vi "Load Core Static.vi"(8 "error in (no error)":errorcluster, 9 "Class Relative Paths Path":path, 10 "Reference Class Path":path, 11 "Message Enqueuer in":refnum<class "Message Enqueuer.lvclass">) -> (0 "error out":errorcluster)   [LabVIEW 2023, in "Class Loader.lvlib" / "Class Loader.lvclass"]
uses:
  Class Loader.lvclass
  Class Loader.lvclass/Class Loader.ctl
  Class Loader Interfaces/Class Loader Interfaces Messages/Class Loading Result Msg/Class Loading Result Msg.lvclass
  eb6241a6-906e-4f6b-ab8e-17d6120ed1e2.vi
  Classes Map.ctl
  <vilib>/ActorFramework/Report Error Msg/Report Error Msg.lvclass
  <vilib>/ActorFramework/Message Enqueuer/Message Enqueuer.lvclass
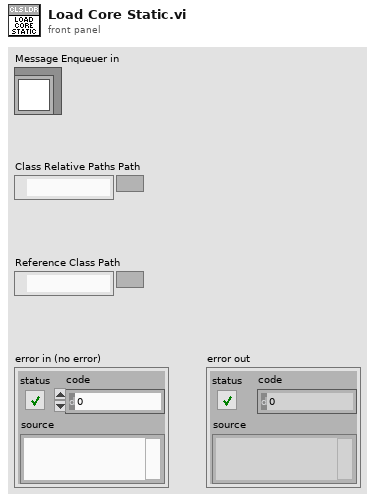
[diagram p1: front panel]
types:
  T1 = typedef "Class Loader.lvlib/Class Loader.lvclass/Classes Map.ctl" = map{string, refnum<class>}
  T2 = typedef "Class Loader.lvlib/Class Loader.lvclass/Class Details.ctl" = cluster{"Class Name":string, "Class":refnum<class>}
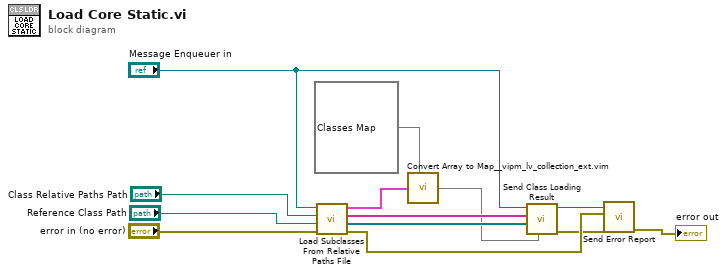
[diagram p0: block diagram]
diagram:
  n1 = call "Load Subclasses From Relative Paths File.vi"("error in"="error in (no error)", "Reference Class Path"="Reference Class Path", "Class Relative Paths Path"="Class Relative Paths Path", "Caller Enqueuer"="Message Enqueuer in") -> ("error out"=w13:errorcluster, "Class Array"=w8:refnum<class>[], "Class Names"=w7:string[], "Class Details Array"=w4:T2[])  [unwired: 4 in]
  n2 = call "Convert Array to Map__vipm_lv_collection_ext.vim"("map type (optional)"=T1 {} ("Classes Map"), "array"=w4) -> ("map"=w6:T1)  [unwired: 5 in]
  n3 = call "Send Class Loading Result.vi"("Classes Map"=w6, "Class Array"=w8, "Class Names"=w7, "Message Enqueuer"="Message Enqueuer in") -> ("error out"=w12:errorcluster, "Message Enqueuer out"=w10:refnum<class "Message Enqueuer.lvclass">)  [unwired: 6 in]
  n4 = call <vilib>:"Send Error Report.vi"("error in (no error)"=w12, "Error From Sender"=w13, "Message Enqueuer"=w10) -> ("error out"=→"error out":errorcluster)  [unwired: 8 in]
